vi "例5-8.vi"() -> ()   [LabVIEW 2019]
uses:
  <vilib>/DAQmx/create/channels.llb/DAQmx Create Channel (CO-Pulse Generation-Frequency).vi
  <vilib>/DAQmx/configure/timing.llb/DAQmx Timing (Implicit).vi
panel:
  in  "停止":bool
  in  "duty cycle":dbl=0.5 caption="占空比" format="%.4f"
  in  "frequency":dbl=1.0 caption="频率" format="%.4f"
  in  "counter":tag caption="计数器"
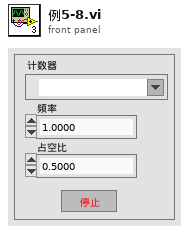
[diagram p1: front panel]
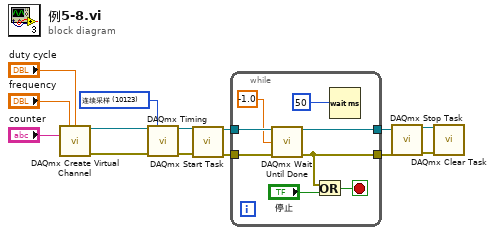
[diagram p0: block diagram]
diagram:
  w9 = 10123 items=["有限采样"=10178, "连续采样"=10123, "硬件定时单点"=12522] ("sample mode")
  n1 = call-poly <vilib>:"DAQmx Create Virtual Channel.vi"("frequency"="frequency", "duty cycle"="duty cycle", "counter"="counter") -> ("task out"=w11:refnum<k21>, "error out"=w10:errorcluster)  [unwired: 11 in]
  n2 = call-poly <vilib>:"DAQmx Timing.vi"("task/channels in"=w11, "sample mode"=w9, "error in"=w10) -> ("task out"=w8:refnum<k21>, "error out"=w7:errorcluster)  [unwired: 11 in]
  n3 = call <vilib>:"DAQmx Start Task.vi"("task/channels in"=w8, "error in"=w7) -> ("task out"=w4:refnum<k21>, "error out"=w3:errorcluster)  [unwired: 12 in]
  n4 = while {
    tunnel: w4 -> [w22]
    tunnel: w3 -> [w21]
    tunnel: [w20] -> w2
    tunnel: [w18] -> w1
    stop <- w16 stop-if-true
    n5 = call <vilib>:"DAQmx Wait Until Done.vi"("task/channels in"=w22, "timeout (sec)"=-1.0, "error in"=w21) -> ("task out"=w20:refnum<k21>, "error out"=w18:errorcluster)  [unwired: 11 in]
    n6 = Or(x=w18, y="停止") -> (x .or. y?=w16:bool)
    n7 = Wait (ms)(milliseconds to wait=50) -> ()  [unwired: 1 out]
  }
  n8 = call <vilib>:"DAQmx Stop Task.vi"("task/channels in"=w2, "error in"=w1) -> ("task out"=w6:refnum<k21>, "error out"=w5:errorcluster)  [unwired: 12 in]
  n9 = call <vilib>:"DAQmx Clear Task.vi"("task in"=w6, "error in"=w5) -> ()  [unwired: 13 in, 1 out]
